vi "Run_Toy_Datasets.vi"(8 "error in (no error)":errorcluster caption="entrée d'erreur (pas d'erreur)", 10 "Fonction":string, 11 "7.2 - Toy datasets en entrée":refnum<class "7.2 - Toy datasets.lvclass">) -> (0 "error out":errorcluster caption="sortie d'erreur", 2 "Out":string, 3 "7.2 - Toy datasets en sortie":refnum<class "7.2 - Toy datasets.lvclass">)   [LabVIEW 2020, in "7.2 - Toy datasets.lvclass"]
uses:
  7.2 - Toy datasets.lvclass
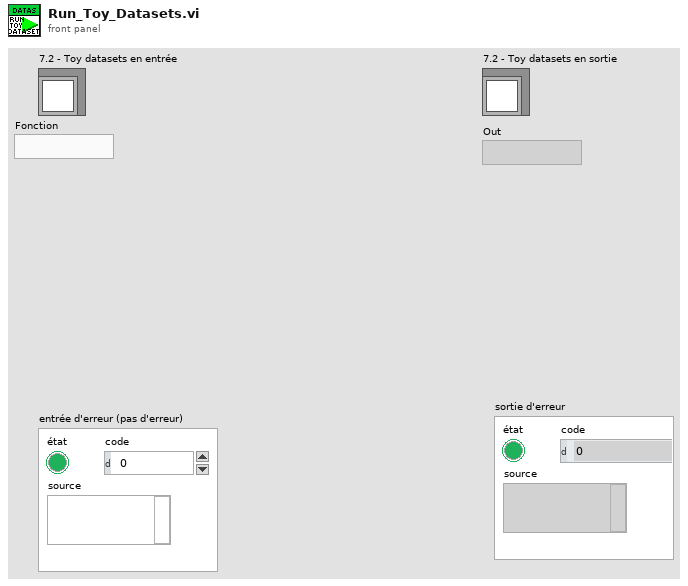
[diagram p1: front panel]
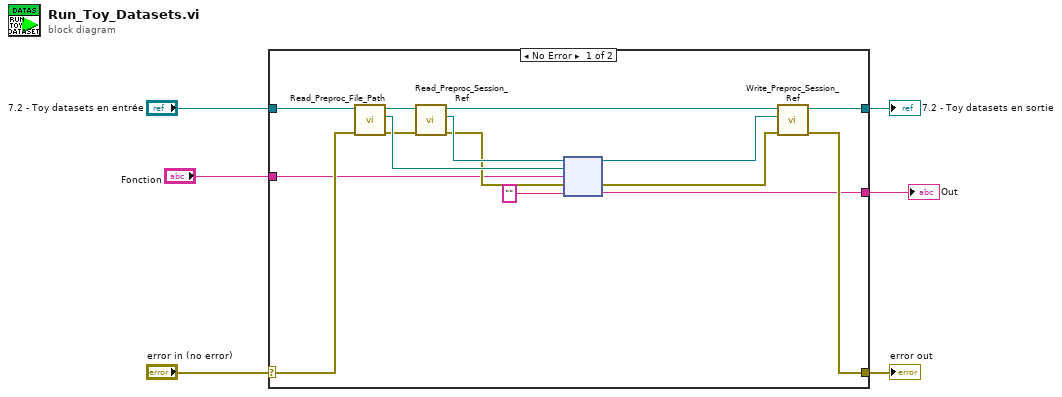
[diagram p0: block diagram]
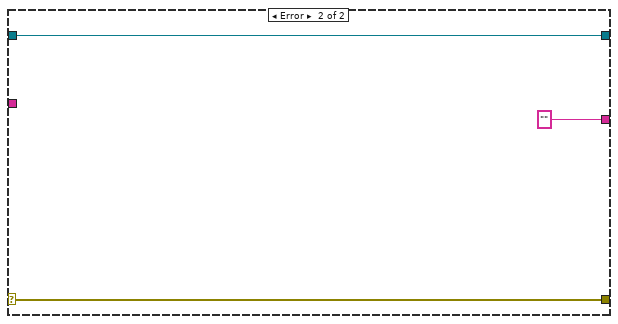
[diagram p2: hidden frame]
diagram:
  n1 = case shown="No Error" "error in (no error)" {
    selector: "error in (no error)" -> [w20 w24]
    tunnel: [w16 w24] -> w5
    tunnel: [w17 w23] -> w3
    tunnel: "7.2 - Toy datasets en entrée" -> [w21 w23]
    tunnel: "Fonction" -> [w9 _]
    tunnel: [w7 ""] -> w1
    frame No Error {
      n2 = call-dynamic "Read_Preproc_File_Path.vi"("error in (no error)"=w20, "Python in"=w21) -> ("error out"=w12:errorcluster, "File_Path"=w15:path, "Python out"=w19:refnum<class "7.2 - Toy datasets.lvclass">)  [unwired: 7 in]
      n3 = call-dynamic "Read_Preproc_Session_Ref.vi"("error in (no error)"=w12, "Python in"=w19) -> ("error out"=w13:errorcluster, "Session_ref"=w14:refnum<k35>, "Python out"=w18:refnum<class "7.2 - Toy datasets.lvclass">)  [unwired: 7 in]
      n4 = node(w14, w15, w9, w13, "") -> (w8:refnum<k35>, w11:errorcluster, w7:string)  [unwired: 2 out]
      n5 = call-dynamic "Write_Preproc_Session_Ref.vi"("error in (no error)"=w11, "Session_ref"=w8, "Python in"=w18) -> ("error out"=w16:errorcluster, "Python out"=w17:refnum<class "7.2 - Toy datasets.lvclass">)  [unwired: 7 in]
    }
    frame Error {
    }
  }
  "error out" <- w5
  "7.2 - Toy datasets en sortie" <- w3
  "Out" <- w1
